vi "nanocal -- nuclear schottky fit V3.vi"() -> ()   [LabVIEW 2020] (continued)
  out "temps&degs":map{i32, map{T1, dbl}}(c390)={4026={enum."T (K)"=0.127, enum."B (T)"=12.0, enum."θ (deg)"=60.0, enum."side (S|R)"=4000.0, enum."change (B|T)"=1.0}, 4027={enum."T (K)"=0.15, enum."B (T)"=12.0, enum."θ (deg)"=60.0, enum."side (S|R)"=4000.0, enum."change (B|T)"=1.0}, 4028={enum."T (K)"=0.179, enum."B (T)"=12.0, enum."θ (deg)"=60.0, enum."side (S|R)"=4000.0, enum."change (B|T)"=1.0}, 4029={enum."T (K)"=0.2, enum."B (T)"=12.0, enum."θ (deg)"=60.0, enum."side (S|R)"=4000.0, enum."change (B|T)"=1.0}, 4030={enum."T (K)"=0.24, enum."B (T)"=12.0, enum."θ (deg)"=60.0, enum."side (S|R)"=4000.0, enum."change (B|T)"=1.0}, 4031={enum."T (K)"=0.287, enum."B (T)"=12.0, enum."θ (deg)"=60.0, enum."side (S|R)"=4000.0, enum."change (B|T)"=1.0}, 4032={enum."T (K)"=0.33, enum."B (T)"=12.0, enum."θ (deg)"=60.0, enum."side (S|R)"=4000.0, enum."change (B|T)"=1.0}, 4033={enum."T (K)"=0.43, enum."B (T)"=12.0, enum."θ (deg)"=60.0, enum."side (S|R)"=4000.0, enum."change (B|T)"=1.0}, 4034={enum."T (K)"=0.51, enum."B (T)"=12.0, enum."θ (deg)"=60.0, enum."side (S|R)"=4000.0, enum."change (B|T)"=1.0}, 4035={enum."T (K)"=0.62, enum."B (T)"=12.0, enum."θ (deg)"=60.0, enum."side (S|R)"=4000.0, enum."change (B|T)"=1.0}, 4036={enum."T (K)"=0.83, enum."B (T)"=12.0, enum."θ (deg)"=60.0, enum."side (S|R)"=4000.0, enum."change (B|T)"=1.0}, 4037={enum."T (K)"=1.13, enum."B (T)"=12.0, enum."θ (deg)"=60.0, enum."side (S|R)"=4000.0, enum."change (B|T)"=1.0}, 4038={enum."T (K)"=1.9, enum."B (T)"=12.0, enum."θ (deg)"=60.0, enum."side (S|R)"=4000.0, enum."change (B|T)"=1.0}, 4039={enum."T (K)"=3.15, enum."B (T)"=12.0, enum."θ (deg)"=60.0, enum."side (S|R)"=4000.0, enum."change (B|T)"=1.0}, 4040={enum."T (K)"=5.7, enum."B (T)"=12.0, enum."θ (deg)"=60.0, enum."side (S|R)"=4000.0, enum."change (B|T)"=1.0}, 4041={enum."T (K)"=7.87, enum."B (T)"=12.0, enum."θ (deg)"=60.0, enum."side (S|R)"=4000.0, enum."change (B|T)"=1.0}, 4042={enum."T (K)"=9.8, enum."B (T)"=12.0, enum."θ (deg)"=60.0, enum."side (S|R)"=4000.0, enum."change (B|T)"=1.0}, 4043={enum."T (K)"=12.36, enum."B (T)"=12.0, enum."θ (deg)"=60.0, enum."side (S|R)"=4000.0, enum."change (B|T)"=1.0}, 4044={enum."T (K)"=14.8, enum."B (T)"=12.0, enum."θ (deg)"=60.0, enum."side (S|R)"=4000.0, enum."change (B|T)"=1.0}, 4045={enum."T (K)"=16.42, enum."B (T)"=12.0, enum."θ (deg)"=60.0, enum."side (S|R)"=4000.0, enum."change (B|T)"=1.0}, 4046={enum."T (K)"=18.04, enum."B (T)"=12.0, enum."θ (deg)"=60.0, enum."side (S|R)"=4000.0, enum."change (B|T)"=1.0}, 4047={enum."T (K)"=0.14, enum."B (T)"=12.0, enum."θ (deg)"=0.0, enum."side (S|R)"=4000.0, enum."change (B|T)"=1.0}, 4048={enum."T (K)"=0.17, enum."B (T)"=12.0, enum."θ (deg)"=0.0, enum."side (S|R)"=4000.0, enum."change (B|T)"=1.0}, 4049={enum."T (K)"=0.2, enum."B (T)"=12.0, enum."θ (deg)"=0.0, enum."side (S|R)"=4000.0, enum."change (B|T)"=1.0}, 4050={enum."T (K)"=0.22, enum."B (T)"=12.0, enum."θ (deg)"=0.0, enum."side (S|R)"=4000.0, enum."change (B|T)"=1.0}, 4051={enum."T (K)"=0.28, enum."B (T)"=12.0, enum."θ (deg)"=0.0, enum."side (S|R)"=4000.0, enum."change (B|T)"=1.0}, 4052={enum."T (K)"=0.33, enum."B (T)"=12.0, enum."θ (deg)"=0.0, enum."side (S|R)"=4000.0, enum."change (B|T)"=1.0}, 4053={enum."T (K)"=0.4, enum."B (T)"=12.0, enum."θ (deg)"=0.0, enum."side (S|R)"=4000.0, enum."change (B|T)"=1.0}, 4054={enum."T (K)"=0.48, enum."B (T)"=12.0, enum."θ (deg)"=0.0, enum."side (S|R)"=4000.0, enum."change (B|T)"=1.0}, 4055={enum."T (K)"=0.58, enum."B (T)"=12.0, enum."θ (deg)"=0.0, enum."side (S|R)"=4000.0, enum."change (B|T)"=1.0}, 4056={enum."T (K)"=0.68, enum."B (T)"=12.0, enum."θ (deg)"=0.0, enum."side (S|R)"=4000.0, enum."change (B|T)"=1.0}, 4057={enum."T (K)"=0.91, enum."B (T)"=12.0, enum."θ (deg)"=0.0, enum."side (S|R)"=4000.0, enum."change (B|T)"=1.0}, 4058={enum."T (K)"=1.23, enum."B (T)"=12.0, enum."θ (deg)"=0.0, enum."side (S|R)"=4000.0, enum."change (B|T)"=1.0}, 4059={enum."T (K)"=1.97, enum."B (T)"=12.0, enum."θ (deg)"=0.0, enum."side (S|R)"=4000.0, enum."change (B|T)"=1.0}, 4060={enum."T (K)"=3.19, enum."B (T)"=12.0, enum."θ (deg)"=0.0, enum."side (S|R)"=4000.0, enum."change (B|T)"=1.0}, 4061={enum."T (K)"=5.82, enum."B (T)"=12.0, enum."θ (deg)"=0.0, enum."side (S|R)"=4000.0, enum."change (B|T)"=1.0}, 4070={enum."T (K)"=0.2, enum."B (T)"=12.0, enum."θ (deg)"=90.0, enum."side (S|R)"=4000.0, enum."change (B|T)"=1.0}, 4071={enum."T (K)"=0.14, enum."B (T)"=12.0, enum."θ (deg)"=90.0, enum."side (S|R)"=4000.0, enum."change (B|T)"=1.0}, 4072={enum."T (K)"=0.18, enum."B (T)"=12.0, enum."θ (deg)"=90.0, enum."side (S|R)"=4000.0, enum."change (B|T)"=1.0}, 4073={enum."T (K)"=0.22, enum."B (T)"=12.0, enum."θ (deg)"=90.0, enum."side (S|R)"=4000.0, enum."change (B|T)"=1.0}, 4074={enum."T (K)"=0.27, enum."B (T)"=12.0, enum."θ (deg)"=90.0, enum."side (S|R)"=4000.0, enum."change (B|T)"=1.0}, 4075={enum."T (K)"=0.33, enum."B (T)"=12.0, enum."θ (deg)"=90.0, enum."side (S|R)"=4000.0, enum."change (B|T)"=1.0}, 4076={enum."T (K)"=0.39, enum."B (T)"=12.0, enum."θ (deg)"=90.0, enum."side (S|R)"=4000.0, enum."change (B|T)"=1.0}, 4077={enum."T (K)"=0.48, enum."B (T)"=12.0, enum."θ (deg)"=90.0, enum."side (S|R)"=4000.0, enum."change (B|T)"=1.0}, 4078={enum."T (K)"=0.58, enum."B (T)"=12.0, enum."θ (deg)"=90.0, enum."side (S|R)"=4000.0, enum."change (B|T)"=1.0}, 4079={enum."T (K)"=0.68, enum."B (T)"=12.0, enum."θ (deg)"=90.0, enum."side (S|R)"=4000.0, enum."change (B|T)"=1.0}, 4080={enum."T (K)"=0.91, enum."B (T)"=12.0, enum."θ (deg)"=90.0, enum."side (S|R)"=4000.0, enum."change (B|T)"=1.0}, 4081={enum."T (K)"=1.23, enum."B (T)"=12.0, enum."θ (deg)"=90.0, enum."side (S|R)"=4000.0, enum."change (B|T)"=1.0}, 4082={enum."T (K)"=2.05, enum."B (T)"=12.0, enum."θ (deg)"=90.0, enum."side (S|R)"=4000.0, enum."change (B|T)"=1.0}, 4083={enum."T (K)"=3.31, enum."B (T)"=12.0, enum."θ (deg)"=90.0, enum."side (S|R)"=4000.0, enum."change (B|T)"=1.0}, 4084={enum."T (K)"=6.0, enum."B (T)"=12.0, enum."θ (deg)"=90.0, enum."side (S|R)"=4000.0, enum."change (B|T)"=1.0}, 4094={enum."T (K)"=0.3, enum."B (T)"=6.0, enum."θ (deg)"=90.0, enum."side (S|R)"=4000.0, enum."change (B|T)"=2.0}, 4095={enum."T (K)"=0.197, enum."B (T)"=6.0, enum."θ (deg)"=90.0, enum."side (S|R)"=4000.0, enum."change (B|T)"=2.0}, 4098={enum."T (K)"=0.148, enum."B (T)"=6.0, enum."θ (deg)"=90.0, enum."side (S|R)"=4000.0, enum."change (B|T)"=2.0}, 4099={enum."T (K)"=0.197, enum."B (T)"=9.0, enum."θ (deg)"=90.0, enum."side (S|R)"=4000.0, enum."change (B|T)"=2.0}, 4100={enum."T (K)"=0.197, enum."B (T)"=11.0, enum."θ (deg)"=90.0, enum."side (S|R)"=4000.0, enum."change (B|T)"=2.0}, 4101={enum."T (K)"=0.197, enum."B (T)"=10.0, enum."θ (deg)"=90.0, enum."side (S|R)"=4000.0, enum."change (B|T)"=2.0}, 4102={enum."T (K)"=0.197, enum."B (T)"=8.0, enum."θ (deg)"=90.0, enum."side (S|R)"=4000.0, enum."change (B|T)"=2.0}, 4103={enum."T (K)"=0.197, enum."B (T)"=7.0, enum."θ (deg)"=90.0, enum."side (S|R)"=4000.0, enum."change (B|T)"=2.0}, 4104={enum."T (K)"=0.197, enum."B (T)"=5.0, enum."θ (deg)"=90.0, enum."side (S|R)"=4000.0, enum."change (B|T)"=2.0}, 4105={enum."T (K)"=0.197, enum."B (T)"=0.0, enum."θ (deg)"=90.0, enum."side (S|R)"=4000.0, enum."change (B|T)"=2.0}, 4106={enum."T (K)"=1.55, enum."B (T)"=0.0, enum."θ (deg)"=90.0, enum."side (S|R)"=4000.0, enum."change (B|T)"=2.0}, 4107={enum."T (K)"=1.0, enum."B (T)"=0.0, enum."θ (deg)"=90.0, enum."side (S|R)"=4000.0, enum."change (B|T)"=2.0}, 4108={enum."T (K)"=0.67, enum."B (T)"=0.0, enum."θ (deg)"=90.0, enum."side (S|R)"=4000.0, enum."change (B|T)"=2.0}, 4110={enum."T (K)"=0.16, enum."B (T)"=12.0, enum."θ (deg)"=30.0, enum."side (S|R)"=4000.0, enum."change (B|T)"=1.0}, 4112={enum."T (K)"=0.17, enum."B (T)"=12.0, enum."θ (deg)"=30.0, enum."side (S|R)"=4000.0, enum."change (B|T)"=1.0}, 4113={enum."T (K)"=0.14, enum."B (T)"=12.0, enum."θ (deg)"=30.0, enum."side (S|R)"=4000.0, enum."change (B|T)"=1.0}, 4114={enum."T (K)"=0.2, enum."B (T)"=12.0, enum."θ (deg)"=30.0, enum."side (S|R)"=4000.0, enum."change (B|T)"=1.0}, 4115={enum."T (K)"=0.25, enum."B (T)"=12.0, enum."θ (deg)"=30.0, enum."side (S|R)"=4000.0, enum."change (B|T)"=1.0}, 4116={enum."T (K)"=0.3, enum."B (T)"=12.0, enum."θ (deg)"=30.0, enum."side (S|R)"=4000.0, enum."change (B|T)"=1.0}, 4117={enum."T (K)"=0.36, enum."B (T)"=12.0, enum."θ (deg)"=30.0, enum."side (S|R)"=4000.0, enum."change (B|T)"=1.0}, 4118={enum."T (K)"=0.43, enum."B (T)"=12.0, enum."θ (deg)"=30.0, enum."side (S|R)"=4000.0, enum."change (B|T)"=1.0}, 4119={enum."T (K)"=0.53, enum."B (T)"=12.0, enum."θ (deg)"=30.0, enum."side (S|R)"=4000.0, enum."change (B|T)"=1.0}, 4120={enum."T (K)"=0.62, enum."B (T)"=12.0, enum."θ (deg)"=30.0, enum."side (S|R)"=4000.0, enum."change (B|T)"=1.0}, 4121={enum."T (K)"=0.83, enum."B (T)"=12.0, enum."θ (deg)"=30.0, enum."side (S|R)"=4000.0, enum."change (B|T)"=1.0}, 4122={enum."T (K)"=1.13, enum."B (T)"=12.0, enum."θ (deg)"=30.0, enum."side (S|R)"=4000.0, enum."change (B|T)"=1.0}, 4123={enum."T (K)"=1.9, enum."B (T)"=12.0, enum."θ (deg)"=30.0, enum."side (S|R)"=4000.0, enum."change (B|T)"=1.0}, 4124={enum."T (K)"=3.1, enum."B (T)"=12.0, enum."θ (deg)"=30.0, enum."side (S|R)"=4000.0, enum."change (B|T)"=1.0}, 8026={enum."T (K)"=0.127, enum."B (T)"=12.0, enum."θ (deg)"=60.0, enum."side (S|R)"=8000.0, enum."change (B|T)"=1.0}, 8027={enum."T (K)"=0.15, enum."B (T)"=12.0, enum."θ (deg)"=60.0, enum."side (S|R)"=8000.0, enum."change (B|T)"=1.0}, 8028={enum."T (K)"=0.179, enum."B (T)"=12.0, enum."θ (deg)"=60.0, enum."side (S|R)"=8000.0, enum."change (B|T)"=1.0}, 8029={enum."T (K)"=0.2, enum."B (T)"=12.0, enum."θ (deg)"=60.0, enum."side (S|R)"=8000.0, enum."change (B|T)"=1.0}, 8030={enum."T (K)"=0.24, enum."B (T)"=12.0, enum."θ (deg)"=60.0, enum."side (S|R)"=8000.0, enum."change (B|T)"=1.0}, 8031={enum."T (K)"=0.287, enum."B (T)"=12.0, enum."θ (deg)"=60.0, enum."side (S|R)"=8000.0, enum."change (B|T)"=1.0}, 8032={enum."T (K)"=0.33, enum."B (T)"=12.0, enum."θ (deg)"=60.0, enum."side (S|R)"=8000.0, enum."change (B|T)"=1.0}, 8033={enum."T (K)"=0.43, enum."B (T)"=12.0, enum."θ (deg)"=60.0, enum."side (S|R)"=8000.0, enum."change (B|T)"=1.0}, 8034={enum."T (K)"=0.51, enum."B (T)"=12.0, enum."θ (deg)"=60.0, enum."side (S|R)"=8000.0, enum."change (B|T)"=1.0}, 8035={enum."T (K)"=0.62, enum."B (T)"=12.0, enum."θ (deg)"=60.0, enum."side (S|R)"=8000.0, enum."change (B|T)"=1.0}, 8036={enum."T (K)"=0.83, enum."B (T)"=12.0, enum."θ (deg)"=60.0, enum."side (S|R)"=8000.0, enum."change (B|T)"=1.0}, 8037={enum."T (K)"=1.13, enum."B (T)"=12.0, enum."θ (deg)"=60.0, enum."side (S|R)"=8000.0, enum."change (B|T)"=1.0}, 8038={enum."T (K)"=1.9, enum."B (T)"=12.0, enum."θ (deg)"=60.0, enum."side (S|R)"=8000.0, enum."change (B|T)"=1.0}, 8039={enum."T (K)"=3.15, enum."B (T)"=12.0, enum."θ (deg)"=60.0, enum."side (S|R)"=8000.0, enum."change (B|T)"=1.0}, 8040={enum."T (K)"=5.7, enum."B (T)"=12.0, enum."θ (deg)"=60.0, enum."side (S|R)"=8000.0, enum."change (B|T)"=1.0}, 8041={enum."T (K)"=7.87, enum."B (T)"=12.0, enum."θ (deg)"=60.0, enum."side (S|R)"=8000.0, enum."change (B|T)"=1.0}, 8042={enum."T (K)"=9.8, enum."B (T)"=12.0, enum."θ (deg)"=60.0, enum."side (S|R)"=8000.0, enum."change (B|T)"=1.0}, 8043={enum."T (K)"=12.36, enum."B (T)"=12.0, enum."θ (deg)"=60.0, enum."side (S|R)"=8000.0, enum."change (B|T)"=1.0}, 8044={enum."T (K)"=14.8, enum."B (T)"=12.0, enum."θ (deg)"=60.0, enum."side (S|R)"=8000.0, enum."change (B|T)"=1.0}, 8045={enum."T (K)"=16.42, enum."B (T)"=12.0, enum."θ (deg)"=60.0, enum."side (S|R)"=8000.0, enum."change (B|T)"=1.0}, 8046={enum."T (K)"=18.04, enum."B (T)"=12.0, enum."θ (deg)"=60.0, enum."side (S|R)"=8000.0, enum."change (B|T)"=1.0}, 8047={enum."T (K)"=0.12, enum."B (T)"=12.0, enum."θ (deg)"=0.0, enum."side (S|R)"=8000.0, enum."change (B|T)"=1.0}, 8048={enum."T (K)"=0.148, enum."B (T)"=12.0, enum."θ (deg)"=0.0, enum."side (S|R)"=8000.0, enum."change (B|T)"=1.0}, 8049={enum."T (K)"=0.179, enum."B (T)"=12.0, enum."θ (deg)"=0.0, enum."side (S|R)"=8000.0, enum."change (B|T)"=1.0}, 8050={enum."T (K)"=0.197, enum."B (T)"=12.0, enum."θ (deg)"=0.0, enum."side (S|R)"=8000.0, enum."change (B|T)"=1.0}, 8051={enum."T (K)"=0.25, enum."B (T)"=12.0, enum."θ (deg)"=0.0, enum."side (S|R)"=8000.0, enum."change (B|T)"=1.0}, 8052={enum."T (K)"=0.3, enum."B (T)"=12.0, enum."θ (deg)"=0.0, enum."side (S|R)"=8000.0, enum."change (B|T)"=1.0}, 8053={enum."T (K)"=0.36, enum."B (T)"=12.0, enum."θ (deg)"=0.0, enum."side (S|R)"=8000.0, enum."change (B|T)"=1.0}, 8054={enum."T (K)"=0.43, enum."B (T)"=12.0, enum."θ (deg)"=0.0, enum."side (S|R)"=8000.0, enum."change (B|T)"=1.0}, 8055={enum."T (K)"=0.512, enum."B (T)"=12.0, enum."θ (deg)"=0.0, enum."side (S|R)"=8000.0, enum."change (B|T)"=1.0}, 8056={enum."T (K)"=0.61, enum."B (T)"=12.0, enum."θ (deg)"=0.0, enum."side (S|R)"=8000.0, enum."change (B|T)"=1.0}, 8057={enum."T (K)"=0.81, enum."B (T)"=12.0, enum."θ (deg)"=0.0, enum."side (S|R)"=8000.0, enum."change (B|T)"=1.0}, 8058={enum."T (K)"=1.12, enum."B (T)"=12.0, enum."θ (deg)"=0.0, enum."side (S|R)"=8000.0, enum."change (B|T)"=1.0}, 8059={enum."T (K)"=1.8, enum."B (T)"=12.0, enum."θ (deg)"=0.0, enum."side (S|R)"=8000.0, enum."change (B|T)"=1.0}, 8060={enum."T (K)"=3.0, enum."B (T)"=12.0, enum."θ (deg)"=0.0, enum."side (S|R)"=8000.0, enum."change (B|T)"=1.0}, 8061={enum."T (K)"=5.5, enum."B (T)"=12.0, enum."θ (deg)"=0.0, enum."side (S|R)"=8000.0, enum."change (B|T)"=1.0}, 8070={enum."T (K)"=0.179, enum."B (T)"=12.0, enum."θ (deg)"=90.0, enum."side (S|R)"=8000.0, enum."change (B|T)"=1.0}, 8071={enum."T (K)"=0.12, enum."B (T)"=12.0, enum."θ (deg)"=90.0, enum."side (S|R)"=8000.0, enum."change (B|T)"=1.0}, 8072={enum."T (K)"=0.148, enum."B (T)"=12.0, enum."θ (deg)"=90.0, enum."side (S|R)"=8000.0, enum."change (B|T)"=1.0}, 8073={enum."T (K)"=0.197, enum."B (T)"=12.0, enum."θ (deg)"=90.0, enum."side (S|R)"=8000.0, enum."change (B|T)"=1.0}, 8074={enum."T (K)"=0.249, enum."B (T)"=12.0, enum."θ (deg)"=90.0, enum."side (S|R)"=8000.0, enum."change (B|T)"=1.0}, 8075={enum."T (K)"=0.3, enum."B (T)"=12.0, enum."θ (deg)"=90.0, enum."side (S|R)"=8000.0, enum."change (B|T)"=1.0}, 8076={enum."T (K)"=0.36, enum."B (T)"=12.0, enum."θ (deg)"=90.0, enum."side (S|R)"=8000.0, enum."change (B|T)"=1.0}, 8077={enum."T (K)"=0.43, enum."B (T)"=12.0, enum."θ (deg)"=90.0, enum."side (S|R)"=8000.0, enum."change (B|T)"=1.0}, 8078={enum."T (K)"=0.512, enum."B (T)"=12.0, enum."θ (deg)"=90.0, enum."side (S|R)"=8000.0, enum."change (B|T)"=1.0}, 8079={enum."T (K)"=0.61, enum."B (T)"=12.0, enum."θ (deg)"=90.0, enum."side (S|R)"=8000.0, enum."change (B|T)"=1.0}, 8080={enum."T (K)"=0.81, enum."B (T)"=12.0, enum."θ (deg)"=90.0, enum."side (S|R)"=8000.0, enum."change (B|T)"=1.0}, 8081={enum."T (K)"=1.1, enum."B (T)"=12.0, enum."θ (deg)"=90.0, enum."side (S|R)"=8000.0, enum."change (B|T)"=1.0}, 8082={enum."T (K)"=1.8, enum."B (T)"=12.0, enum."θ (deg)"=90.0, enum."side (S|R)"=8000.0, enum."change (B|T)"=1.0}, 8083={enum."T (K)"=3.0, enum."B (T)"=12.0, enum."θ (deg)"=90.0, enum."side (S|R)"=8000.0, enum."change (B|T)"=1.0}, 8084={enum."T (K)"=5.7, enum."B (T)"=12.0, enum."θ (deg)"=90.0, enum."side (S|R)"=8000.0, enum."change (B|T)"=1.0}, 8094={enum."T (K)"=0.3, enum."B (T)"=6.0, enum."θ (deg)"=90.0, enum."side (S|R)"=8000.0, enum."change (B|T)"=2.0}, 8095={enum."T (K)"=0.197, enum."B (T)"=6.0, enum."θ (deg)"=90.0, enum."side (S|R)"=8000.0, enum."change (B|T)"=2.0}, 8098={enum."T (K)"=0.148, enum."B (T)"=6.0, enum."θ (deg)"=90.0, enum."side (S|R)"=8000.0, enum."change (B|T)"=2.0}, 8099={enum."T (K)"=0.197, enum."B (T)"=9.0, enum."θ (deg)"=90.0, enum."side (S|R)"=8000.0, enum."change (B|T)"=2.0}, 8100={enum."T (K)"=0.197, enum."B (T)"=11.0, enum."θ (deg)"=90.0, enum."side (S|R)"=8000.0, enum."change (B|T)"=2.0}, 8101={enum."T (K)"=0.197, enum."B (T)"=10.0, enum."θ (deg)"=90.0, enum."side (S|R)"=8000.0, enum."change (B|T)"=2.0}, 8102={enum."T (K)"=0.197, enum."B (T)"=8.0, enum."θ (deg)"=90.0, enum."side (S|R)"=8000.0, enum."change (B|T)"=2.0}, 8103={enum."T (K)"=0.197, enum."B (T)"=7.0, enum."θ (deg)"=90.0, enum."side (S|R)"=8000.0, enum."change (B|T)"=2.0}, 8104={enum."T (K)"=0.197, enum."B (T)"=5.0, enum."θ (deg)"=90.0, enum."side (S|R)"=8000.0, enum."change (B|T)"=2.0}, 8105={enum."T (K)"=0.197, enum."B (T)"=0.0, enum."θ (deg)"=90.0, enum."side (S|R)"=8000.0, enum."change (B|T)"=2.0}, 8106={enum."T (K)"=1.55, enum."B (T)"=0.0, enum."θ (deg)"=90.0, enum."side (S|R)"=8000.0, enum."change (B|T)"=2.0}, 8107={enum."T (K)"=1.0, enum."B (T)"=0.0, enum."θ (deg)"=90.0, enum."side (S|R)"=8000.0, enum."change (B|T)"=2.0}, 8108={enum."T (K)"=0.67, enum."B (T)"=0.0, enum."θ (deg)"=90.0, enum."side (S|R)"=8000.0, enum."change (B|T)"=2.0}, 8110={enum."T (K)"=0.16, enum."B (T)"=12.0, enum."θ (deg)"=30.0, enum."side (S|R)"=8000.0, enum."change (B|T)"=1.0}, 8112={enum."T (K)"=0.17, enum."B (T)"=12.0, enum."θ (deg)"=30.0, enum."side (S|R)"=8000.0, enum."change (B|T)"=1.0}, 8113={enum."T (K)"=0.14, enum."B (T)"=12.0, enum."θ (deg)"=30.0, enum."side (S|R)"=8000.0, enum."change (B|T)"=1.0}, 8114={enum."T (K)"=0.2, enum."B (T)"=12.0, enum."θ (deg)"=30.0, enum."side (S|R)"=8000.0, enum."change (B|T)"=1.0}, 8115={enum."T (K)"=0.25, enum."B (T)"=12.0, enum."θ (deg)"=30.0, enum."side (S|R)"=8000.0, enum."change (B|T)"=1.0}, 8116={enum."T (K)"=0.3, enum."B (T)"=12.0, enum."θ (deg)"=30.0, enum."side (S|R)"=8000.0, enum."change (B|T)"=1.0}, 8117={enum."T (K)"=0.36, enum."B (T)"=12.0, enum."θ (deg)"=30.0, enum."side (S|R)"=8000.0, enum."change (B|T)"=1.0}, 8118={enum."T (K)"=0.43, enum."B (T)"=12.0, enum."θ (deg)"=30.0, enum."side (S|R)"=8000.0, enum."change (B|T)"=1.0}, 8119={enum."T (K)"=0.53, enum."B (T)"=12.0, enum."θ (deg)"=30.0, enum."side (S|R)"=8000.0, enum."change (B|T)"=1.0}, 8120={enum."T (K)"=0.62, enum."B (T)"=12.0, enum."θ (deg)"=30.0, enum."side (S|R)"=8000.0, enum."change (B|T)"=1.0}, 8121={enum."T (K)"=0.83, enum."B (T)"=12.0, enum."θ (deg)"=30.0, enum."side (S|R)"=8000.0, enum."change (B|T)"=1.0}, 8122={enum."T (K)"=1.13, enum."B (T)"=12.0, enum."θ (deg)"=30.0, enum."side (S|R)"=8000.0, enum."change (B|T)"=1.0}, 8123={enum."T (K)"=1.9, enum."B (T)"=12.0, enum."θ (deg)"=30.0, enum."side (S|R)"=8000.0, enum."change (B|T)"=1.0}, 8124={enum."T (K)"=3.1, enum."B (T)"=12.0, enum."θ (deg)"=30.0, enum."side (S|R)"=8000.0, enum."change (B|T)"=1.0}, 40047={enum."T (K)"=19.6, enum."B (T)"=12.0, enum."θ (deg)"=60.0, enum."side (S|R)"=4000.0, enum."change (B|T)"=1.0}, 40049={enum."T (K)"=0.129, enum."B (T)"=12.0, enum."θ (deg)"=60.0, enum."side (S|R)"=4000.0, enum."change (B|T)"=1.0}, 40125={enum."T (K)"=0.157, enum."B (T)"=12.0, enum."θ (deg)"=45.0, enum."side (S|R)"=4000.0, enum."change (B|T)"=1.0}, 40126={enum."T (K)"=0.12, enum."B (T)"=12.0, enum."θ (deg)"=45.0, enum."side (S|R)"=4000.0, enum."change (B|T)"=1.0}, 40127={enum."T (K)"=0.17, enum."B (T)"=12.0, enum."θ (deg)"=45.0, enum."side (S|R)"=4000.0, enum."change (B|T)"=1.0}, 40128={enum."T (K)"=0.2, enum."B (T)"=12.0, enum."θ (deg)"=45.0, enum."side (S|R)"=4000.0, enum."change (B|T)"=1.0}, 40129={enum."T (K)"=0.255, enum."B (T)"=12.0, enum."θ (deg)"=45.0, enum."side (S|R)"=4000.0, enum."change (B|T)"=1.0}, 40130={enum."T (K)"=0.3, enum."B (T)"=12.0, enum."θ (deg)"=45.0, enum."side (S|R)"=4000.0, enum."change (B|T)"=1.0}, 40131={enum."T (K)"=0.36, enum."B (T)"=12.0, enum."θ (deg)"=45.0, enum."side (S|R)"=4000.0, enum."change (B|T)"=1.0}, 40132={enum."T (K)"=0.43, enum."B (T)"=12.0, enum."θ (deg)"=45.0, enum."side (S|R)"=4000.0, enum."change (B|T)"=1.0}, 40133={enum."T (K)"=0.53, enum."B (T)"=12.0, enum."θ (deg)"=45.0, enum."side (S|R)"=4000.0, enum."change (B|T)"=1.0}, 40134={enum."T (K)"=0.62, enum."B (T)"=12.0, enum."θ (deg)"=45.0, enum."side (S|R)"=4000.0, enum."change (B|T)"=1.0}, 40135={enum."T (K)"=0.83, enum."B (T)"=12.0, enum."θ (deg)"=45.0, enum."side (S|R)"=4000.0, enum."change (B|T)"=1.0}, 40136={enum."T (K)"=1.13, enum."B (T)"=12.0, enum."θ (deg)"=45.0, enum."side (S|R)"=4000.0, enum."change (B|T)"=1.0}, 40137={enum."T (K)"=1.9, enum."B (T)"=12.0, enum."θ (deg)"=45.0, enum."side (S|R)"=4000.0, enum."change (B|T)"=1.0}, 40138={enum."T (K)"=3.1, enum."B (T)"=12.0, enum."θ (deg)"=45.0, enum."side (S|R)"=4000.0, enum."change (B|T)"=1.0}, 40139={enum."T (K)"=5.7, enum."B (T)"=12.0, enum."θ (deg)"=45.0, enum."side (S|R)"=4000.0, enum."change (B|T)"=1.0}, 80047={enum."T (K)"=19.6, enum."B (T)"=12.0, enum."θ (deg)"=60.0, enum."side (S|R)"=8000.0, enum."change (B|T)"=1.0}, 80049={enum."T (K)"=0.129, enum."B (T)"=12.0, enum."θ (deg)"=60.0, enum."side (S|R)"=8000.0, enum."change (B|T)"=1.0}, 80125={enum."T (K)"=0.157, enum."B (T)"=12.0, enum."θ (deg)"=45.0, enum."side (S|R)"=8000.0, enum."change (B|T)"=1.0}, 80126={enum."T (K)"=0.12, enum."B (T)"=12.0, enum."θ (deg)"=45.0, enum."side (S|R)"=8000.0, enum."change (B|T)"=1.0}, 80127={enum."T (K)"=0.17, enum."B (T)"=12.0, enum."θ (deg)"=45.0, enum."side (S|R)"=8000.0, enum."change (B|T)"=1.0}, 80128={enum."T (K)"=0.2, enum."B (T)"=12.0, enum."θ (deg)"=45.0, enum."side (S|R)"=8000.0, enum."change (B|T)"=1.0}, 80129={enum."T (K)"=0.255, enum."B (T)"=12.0, enum."θ (deg)"=45.0, enum."side (S|R)"=8000.0, enum."change (B|T)"=1.0}, 80130={enum."T (K)"=0.3, enum."B (T)"=12.0, enum."θ (deg)"=45.0, enum."side (S|R)"=8000.0, enum."change (B|T)"=1.0}, 80131={enum."T (K)"=0.36, enum."B (T)"=12.0, enum."θ (deg)"=45.0, enum."side (S|R)"=8000.0, enum."change (B|T)"=1.0}, 80132={enum."T (K)"=0.43, enum."B (T)"=12.0, enum."θ (deg)"=45.0, enum."side (S|R)"=8000.0, enum."change (B|T)"=1.0}, 80133={enum."T (K)"=0.53, enum."B (T)"=12.0, enum."θ (deg)"=45.0, enum."side (S|R)"=8000.0, enum."change (B|T)"=1.0}, 80134={enum."T (K)"=0.62, enum."B (T)"=12.0, enum."θ (deg)"=45.0, enum."side (S|R)"=8000.0, enum."change (B|T)"=1.0}, 80135={enum."T (K)"=0.83, enum."B (T)"=12.0, enum."θ (deg)"=45.0, enum."side (S|R)"=8000.0, enum."change (B|T)"=1.0}, 80136={enum."T (K)"=1.13, enum."B (T)"=12.0, enum."θ (deg)"=45.0, enum."side (S|R)"=8000.0, enum."change (B|T)"=1.0}, 80137={enum."T (K)"=1.9, enum."B (T)"=12.0, enum."θ (deg)"=45.0, enum."side (S|R)"=8000.0, enum."change (B|T)"=1.0}, 80138={enum."T (K)"=3.1, enum."B (T)"=12.0, enum."θ (deg)"=45.0, enum."side (S|R)"=8000.0, enum."change (B|T)"=1.0}, 80139={enum."T (K)"=5.7, enum."B (T)"=12.0, enum."θ (deg)"=45.0, enum."side (S|R)"=8000.0, enum."change (B|T)"=1.0}}
  out "mathematica thing":map{i32, map{T1, dbl}}(c390)
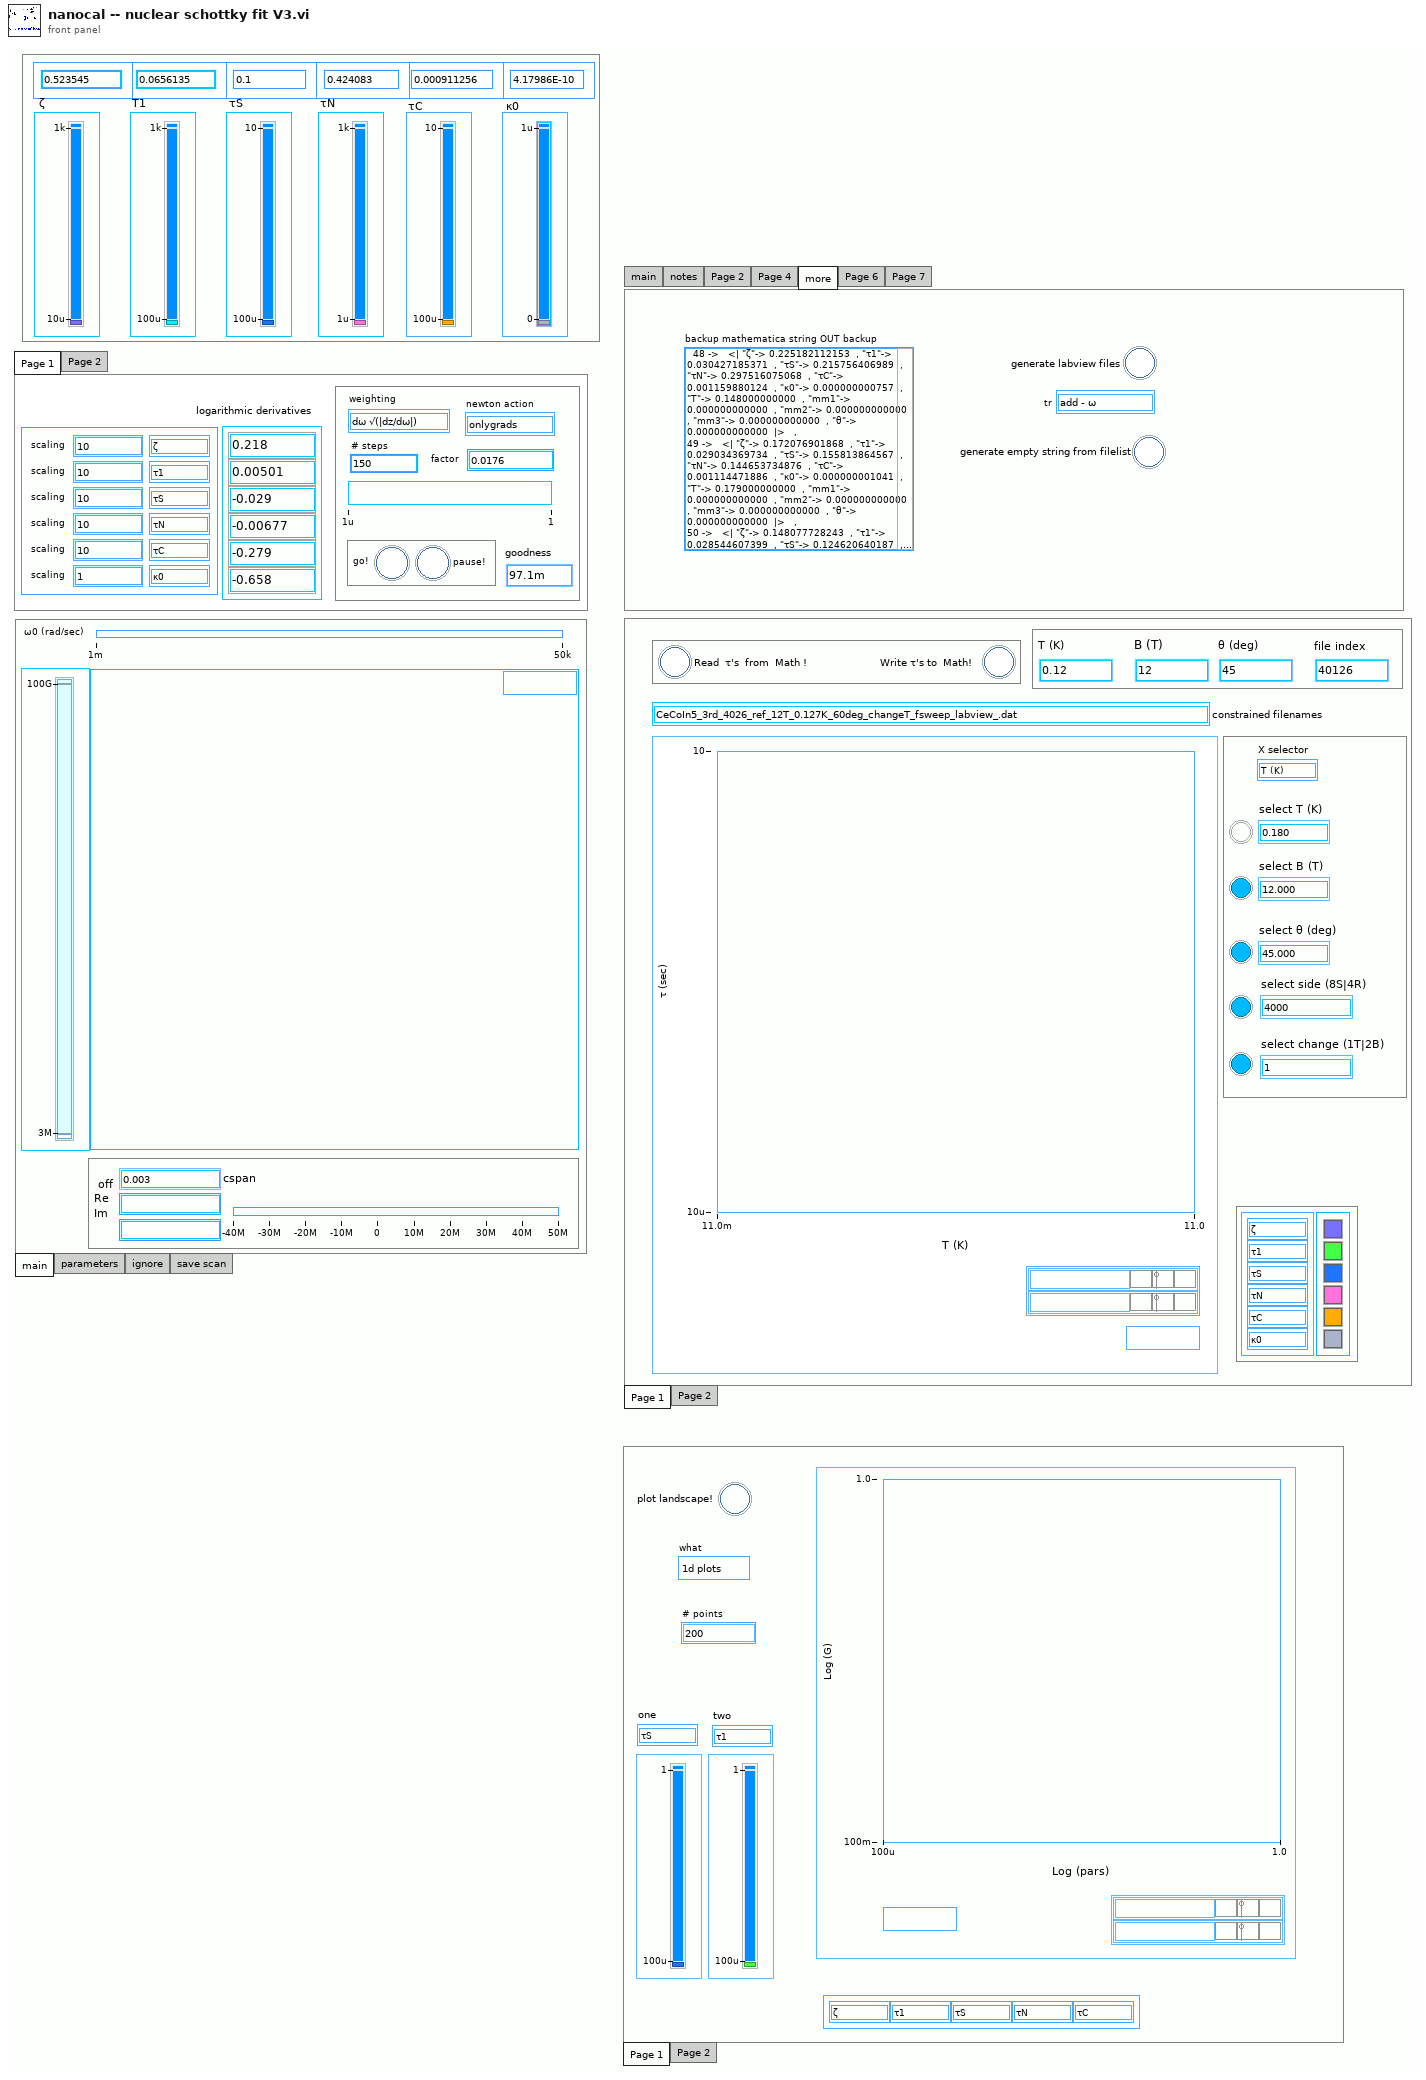
[diagram p1: front panel]
types:
  T1 = typedef "3-lorentzian-parameters.ctl" = enum16{"ζ", "τ1", "τS", "τN", "τC", "κ0", "m1", "m2", "m3", "T (K)", "B (T)", "θ (deg)", "side (S|R)", "change (B|T)"}
  T2 = enum32{"main", "notes", "Page 2", "Page 4", "more", "Page 6", "Page 7"}
  T3 = typedef "nanocal_data_read_format.ctl" = enum16{"as is", "add - ω", "full rydh", "raw nanocal"}
